vi "GET_Index_of_selected_Tree_element_and_N_Conditions.vi"(8 "error in (no error)":errorcluster, 11 "TreeControl in":refnum<vi>) -> (0 "error out":errorcluster, 1 "Index of selected element":i32, 2 "Amount of conditions":i32, 3 "TreeControl out":refnum<vi>)   [LabVIEW 2018, in "Tracker.lvlib"]
uses:
  Tracker.lvlib
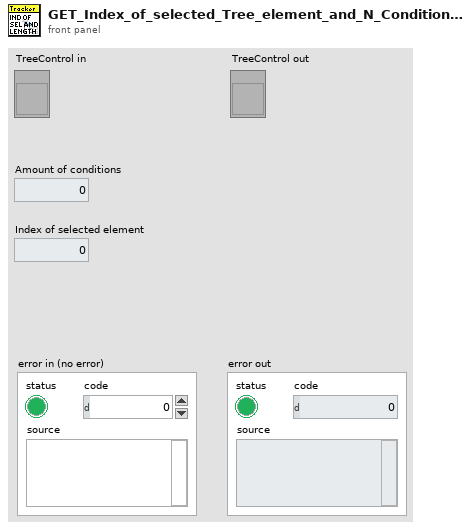
[diagram p1: front panel]
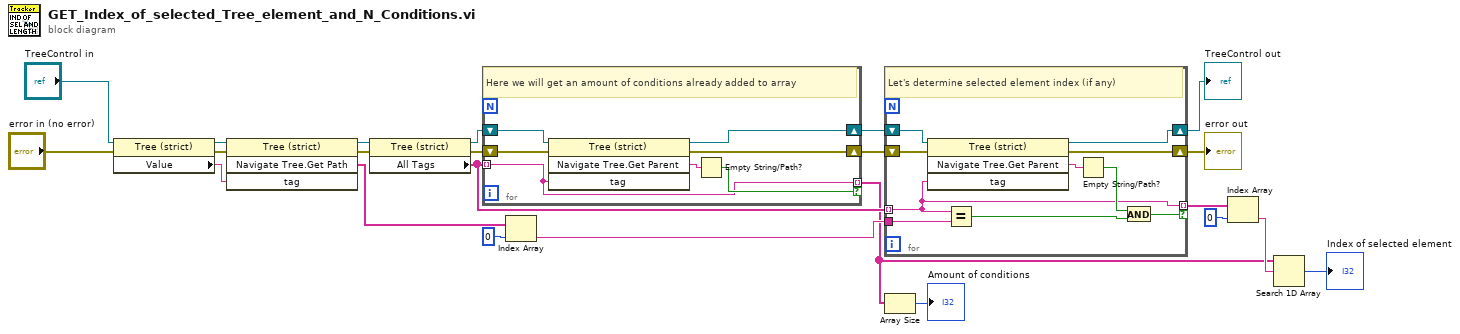
[diagram p0: block diagram]
diagram:
  n1 = property class="Tree (strict)"(reference="TreeControl in", error in="error in (no error)") -> (reference out=w16:refnum<vi>, error out=w17:errorcluster, "Value"=w15:string)
  n2 = invoke class="Tree (strict)" method="Navigate Tree.Get Path"(reference=w16, error in=w17, "tag"=w15) -> (reference out=w13:refnum<vi>, error out=w12:errorcluster, "Navigate Tree:Get Path"=w14:string[])  [unwired: 1 in, 1 out]
  n3 = property class="Tree (strict)"(reference=w13, error in=w12) -> (reference out=w8:refnum<vi>, error out=w7:errorcluster, "All Tags"=w6:string[])
  n4 = for {
    tunnel: w6 -> [w24] mode=indexing
    tunnel: [w24] -> w2 mode=indexing if=w29
    shift-right: [w26] -> w4
    shift-left: w7 -> [w28]
    shift-right: [w27] -> w3
    shift-left: w8 -> [w25]
    # "Here we will get an amount of conditions already added to array"
    n5 = invoke class="Tree (strict)" method="Navigate Tree.Get Parent"(reference=w25, error in=w28, "tag"=w24) -> (reference out=w27:refnum<vi>, error out=w26:errorcluster, "Navigate Tree:Get Parent"=w30:string)  [unwired: 1 in, 1 out]
    n6 = Empty String/Path?(string/path=w30) -> (empty?=w29:bool)
  }
  n7 = Index Array(array=w14, index=0) -> (element=w5:string)
  n8 = for {
    tunnel: w6 -> [w31] mode=indexing
    tunnel: [w31] -> w20 mode=indexing if=w33
    shift-right: [w36] -> w19
    shift-left: w4 -> [w38]
    shift-right: [w37] -> w18
    shift-left: w3 -> [w35]
    tunnel: w5 -> [w34]
    # "Let's determine selected element index (if any)"
    n9 = invoke class="Tree (strict)" method="Navigate Tree.Get Parent"(reference=w35, error in=w38, "tag"=w31) -> (reference out=w37:refnum<vi>, error out=w36:errorcluster, "Navigate Tree:Get Parent"=w40:string)  [unwired: 1 in, 1 out]
    n10 = Equal?(x=w31, y=w34) -> (x = y?=w32:bool)
    n11 = Empty String/Path?(string/path=w40) -> (empty?=w39:bool)
    n12 = And(x=w39, y=w32) -> (x .and. y?=w33:bool)
  }
  "error out" <- w19
  "TreeControl out" <- w18
  n13 = Array Size(array=w2) -> (size(s)=→"Amount of conditions":i32)
  n14 = Index Array(array=w20, index=0) -> (element=w21:string)
  n15 = Search 1D Array(1D array=w2, element=w21) -> (index of element=→"Index of selected element":i32)  [unwired: 1 in]
